vi "GetInputConfiguration.vi"(11 "Properties":T2[](array[typedef])) -> (3 "Input Configuration":T1 items=["AC Coupled", "DC Coupled", "IEPE AC Coupled"])   [LabVIEW 2017, in "CmsAcquisition.lvlib"]
uses:
  <vilib>/addons/InsightCM/Devices/Shared/Cms/CmsAcquisition/CmsAcquisition.lvlib
  <vilib>/addons/InsightCM/MessageBus/Base/controls/KeyValuePair.ctl
  <vilib>/LabVIEW Targets/FPGA/cRIO/shared/nicrio_ModuleControls/nicrio_cRIO-9232_ConfigModeRing.ctl
  <vilib>/addons/InsightCM/Utilities/PropertyHelpers/PropertyHelpers.lvlib
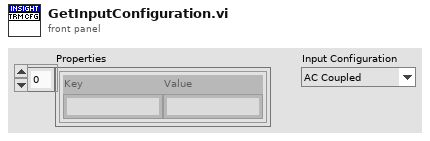
[diagram p1: front panel]
types:
  T1 = typedef "nicrio_cRIO-9232_ConfigModeRing.ctl" = u8
  T2 = typedef "KeyValuePair.ctl" = cluster{"Key":string, "Value":string}
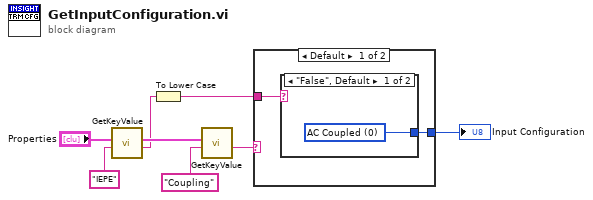
[diagram p0: block diagram]
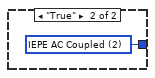
[diagram p2: hidden frame]
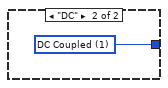
[diagram p3: hidden frame]
diagram:
  n1 = call <vilib>:"GetKeyValue.vi"("key"="IEPE" ("name"), "key value pairs"="Properties") -> ("value"=w3:string, "key value pairs out"=w5:T2[])  [unwired: 7 in, 1 out]
  n2 = To Lower Case(string=w3) -> (all lower case string=w8:string)
  n3 = call <vilib>:"GetKeyValue.vi"("key"="Coupling" ("name"), "key value pairs"=w5) -> ("value"=w1:string)  [unwired: 7 in, 2 out]
  n4 = case shown="Default" w1 {
    tunnel: w8 -> [w10 _]
    tunnel: [w9 w13] -> w7
    frame Default {
      n5 = case shown="\"False\", Default" w10 {
        tunnel: [w11 w12] -> w9
        frame "False", Default {
          w11 = T1 0 items=["AC Coupled", "DC Coupled", "IEPE AC Coupled"] ("Input_Configuration")
        }
        frame "True" {
          w12 = T1 2 items=["AC Coupled", "DC Coupled", "IEPE AC Coupled"] ("Input_Configuration")
        }
      }
    }
    frame "DC" {
      w13 = T1 1 items=["AC Coupled", "DC Coupled", "IEPE AC Coupled"] ("Input_Configuration")
    }
  }
  "Input Configuration" <- w7
